vi "MC-21C Driver_query.vi"(0 "Peristaltic Pump COM":refnum<visa-resource-name>="COM3", 1 "Speed (rpm)":string, 5 "Operation":T1(ring), 7 "Address":u8, 9 "Set address (0-255)":u8, 12 "Step":string) -> (6 "PerisPump running":bool, 10 "Write buffer":string, 15 "Read buffer":string)   [LabVIEW 2023]
panel:
  out "Current address":u8
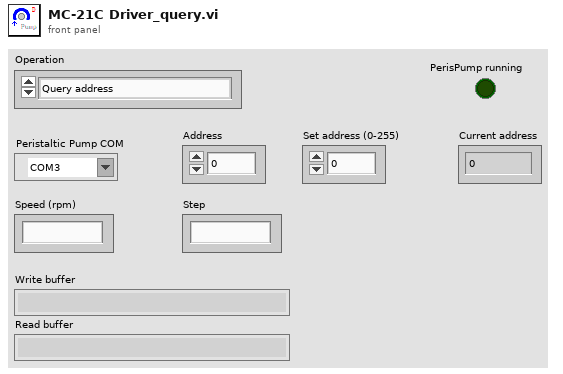
[diagram p1: front panel]
types:
  T1 = enum16{"Query address", "Set address", "Set speed", "Clockwise rotation", "Counterclockwise rotation", "Stop"}
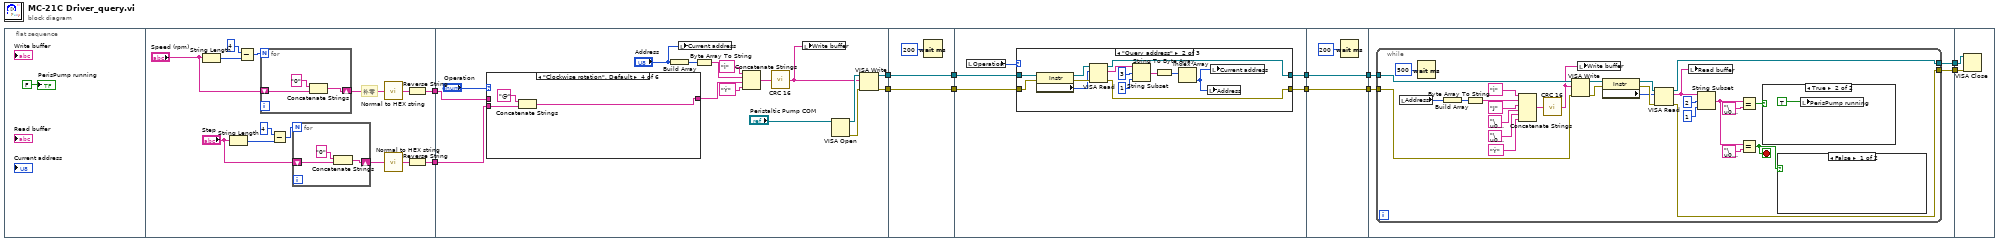
[diagram p0: block diagram]
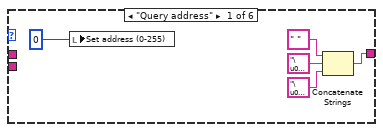
[diagram p2: hidden frame]
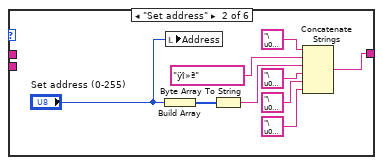
[diagram p3: hidden frame]
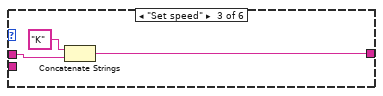
[diagram p4: hidden frame]
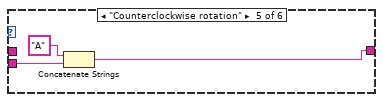
[diagram p5: hidden frame]
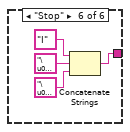
[diagram p6: hidden frame]
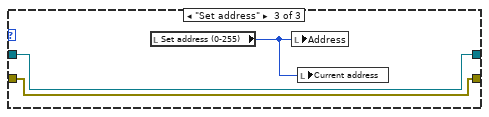
[diagram p8: hidden frame]
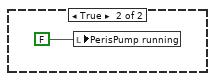
[diagram p10: hidden frame]
diagram:
  n1 = flat-sequence {
    tunnel: [w21] -> w11
    tunnel: [w14] -> w12
    tunnel: [w42] -> w6
    tunnel: [w41] -> w4
    tunnel: w12 -> [w40]
    tunnel: w11 -> [w39]
    tunnel: w6 -> [w79]
    tunnel: [w79] -> w5
    tunnel: w4 -> [w78]
    tunnel: [w78] -> w3
    tunnel: w5 -> [w83]
    tunnel: [w81] -> w8
    tunnel: w3 -> [w82]
    tunnel: [w80] -> w7
    tunnel: w8 -> [w105]
    tunnel: [w105] -> w10
    tunnel: w7 -> [w104]
    tunnel: [w104] -> w9
    tunnel: w10 -> [w109]
    tunnel: w9 -> [w108]
    tunnel: [w107] -> w2
    tunnel: [w106] -> w1
    tunnel: w2 -> [w141]
    tunnel: w1 -> [w140]
    frame #0 {
      "PerisPump running" <- FALSE ("PerisPump running")
    }
    frame #1 {
      # "补零"
      n2 = String Length(string="Speed (rpm)") -> (length=w25:i32)
      n3 = String Length(string="Step") -> (length=w19:i32)
      n4 = Subtract(x=4, y=w25) -> (x-y=w27:i32)
      n5 = for {
        N: w27 -> [_]
        shift-right: [w31] -> w23
        shift-left: "Speed (rpm)" -> [w33]
        n6 = Concatenate Strings("0" ("string"), w33) -> (w31:string)
      }
      n7 = Subtract(x=4, y=w19) -> (x-y=w18:i32)
      n8 = for {
        N: w18 -> [_]
        shift-right: [w28] -> w16
        shift-left: "Step" -> [w30]
        n9 = Concatenate Strings("0" ("string"), w30) -> (w28:string)
      }
      n10 = call "Normal to HEX string.vi"("input normal string"=w23) -> ("output HEX string"=w22:string)
      n11 = call "Normal to HEX string.vi"("input normal string"=w16) -> ("output HEX string"=w20:string)
      n12 = Reverse String(1:w22) -> (0:w21:string)
      n13 = Reverse String(1:w20) -> (0:w14:string)
    }
    frame #2 {
      n14 = case shown="\"Clockwise rotation\", Default" "Operation" {
        tunnel: [w50 w58 w65 w68 w71 w73] -> w46
        tunnel: w40 -> [_ _ _ w67 w70 _]
        tunnel: w39 -> [_ _ w64 _ _ _]
        frame "Query address" {
          n15 = local write "Set address (0-255)"(u8 0 ("Address (0-255)")) -> ()
          n16 = Concatenate Strings(" " ("string"), "\u0000" ("string"), "\u0000" ("string")) -> (w50:string)
        }
        frame "Set address" {
          n17 = Build Array("Set address (0-255)") -> (w57:u8[])
          n18 = local write "Address"("Set address (0-255)") -> ()
          n19 = Byte Array To String(unsigned byte array=w57) -> (string=w56:string)
          n20 = Concatenate Strings("\u0000" ("string"), "ÿî»ª" ("string"), w56, "\u0000" ("string"), "\u0000" ("string"), "\u0000" ("string")) -> (w58:string)
        }
        frame "Set speed" {
          n21 = Concatenate Strings("K" ("string"), w64) -> (w65:string)
        }
        frame "Clockwise rotation", Default {
          n22 = Concatenate Strings("@" ("string"), w67) -> (w68:string)
        }
        frame "Counterclockwise rotation" {
          n23 = Concatenate Strings("A" ("string"), w70) -> (w71:string)
        }
        frame "Stop" {
          n24 = Concatenate Strings("I" ("string"), "\u0000" ("string"), "\u0000" ("string")) -> (w73:string)
        }
      }
      n25 = Build Array("Address") -> (w38:u8[])
      n26 = local write "Current address"("Address") -> ()
      n27 = Byte Array To String(unsigned byte array=w38) -> (string=w37:string)
      n28 = Concatenate Strings("Ì" ("string"), w37, w46, "Ý" ("string")) -> (w36:string)
      n29 = call "CRC 16.vi"("input HEX string"=w36) -> ("output HEX string"=w35:string)
      n30 = local write "Write buffer"(w35) -> ()
      n31 = VISA Open(VISA resource name="Peristaltic Pump COM") -> (VISA resource name=w45:refnum<visa-resource-name>, error out=w44:errorcluster)  [unwired: 4 in]
      n32 = VISA Write(VISA resource name=w45, write buffer=w35, error in (no error)=w44) -> (VISA resource name out=w42:refnum<visa-resource-name>, error out=w41:errorcluster)  [unwired: 1 out]
    }
    frame #3 {
      n33 = Wait (ms)(milliseconds to wait=u32 200) -> ()  [unwired: 1 out]
    }
    frame #4 {
      n34 = local read "Operation"() -> (w84:T1)
      n35 = case shown="\"Query address\"" w84 {
        tunnel: w83 -> [w86 w96 w102]
        tunnel: w82 -> [w85 w95 w101]
        tunnel: [w86 w89 w102] -> w81
        tunnel: [w85 w88 w101] -> w80
        frame "Set speed", Default {
        }
        frame "Query address" {
          n36 = property class="Instr"(reference=w96, error in=w95) -> (reference out=w99:refnum<visa-resource-name>, error out=w98:errorcluster, "Serial Settings:Number of Bytes at Serial Port"=w97:u32)
          n37 = VISA Read(VISA resource name=w99, byte count=w97, error in (no error)=w98) -> (VISA resource name out=w89:refnum<visa-resource-name>, read buffer=w92:string, error out=w88:errorcluster)  [unwired: 1 out]
          n38 = String Subset(string=w92, offset (0)=3, length (rest)=1 ("length (rest)")) -> (substring=w91:string)
          n39 = String To Byte Array(string=w91) -> (unsigned byte array=w90:u8[])
          n40 = Index Array(array=w90) -> (element=w87:u8)  [unwired: 1 in]
          n41 = local write "Address"(w87) -> ()
          n42 = local write "Current address"(w87) -> ()
        }
        frame "Set address" {
          n43 = local read "Set address (0-255)"() -> (w100:u8)
          n44 = local write "Address"(w100) -> ()
          n45 = local write "Current address"(w100) -> ()
        }
      }
    }
    frame #5 {
      n46 = Wait (ms)(milliseconds to wait=u32 200) -> ()  [unwired: 1 out]
    }
    frame #6 {
      n47 = while {
        tunnel: w109 -> [w128]
        tunnel: w108 -> [w127]
        tunnel: [w124] -> w107
        tunnel: [w123] -> w106
        stop <- w114 stop-if-true
        n48 = local read "Address"() -> (w132:u8)
        n49 = Wait (ms)(milliseconds to wait=u32 500) -> ()  [unwired: 1 out]
        n50 = Build Array(w132) -> (w133:u8[])
        n51 = Byte Array To String(unsigned byte array=w133) -> (string=w131:string)
        n52 = Concatenate Strings("Ì" ("string"), w131, "J" ("string"), "\u0000" ("string"), "\u0000" ("string"), "Ý" ("string")) -> (w117:string)
        n53 = call "CRC 16.vi"("input HEX string"=w117) -> ("output HEX string"=w116:string)
        n54 = VISA Write(VISA resource name=w128, write buffer=w116, error in (no error)=w127) -> (VISA resource name out=w122:refnum<visa-resource-name>, error out=w121:errorcluster)  [unwired: 1 out]
        n55 = local write "Write buffer"(w116) -> ()
        n56 = property class="Instr"(reference=w122, error in=w121) -> (reference out=w120:refnum<visa-resource-name>, error out=w119:errorcluster, "Serial Settings:Number of Bytes at Serial Port"=w118:u32)
        n57 = VISA Read(VISA resource name=w120, byte count=w118, error in (no error)=w119) -> (VISA resource name out=w124:refnum<visa-resource-name>, read buffer=w115:string, error out=w123:errorcluster)  [unwired: 1 out]
        n58 = local write "Read buffer"(w115) -> ()
        n59 = String Subset(string=w115, offset (0)=2, length (rest)=1 ("length (rest)")) -> (substring=w112:string)
        n60 = Equal?(x=w112, y="\u0004") -> (x = y?=w110:bool)
        n61 = Equal?(x=w112, y="\u0000") -> (x = y?=w114:bool)
        n62 = case shown="True" w110 {
          frame False {
          }
          frame True {
            n63 = local write "PerisPump running"(TRUE ("PerisPump running")) -> ()
          }
        }
        n64 = case shown="False" w114 {
          frame False {
          }
          frame True {
            n65 = local write "PerisPump running"(FALSE ("PerisPump running")) -> ()
          }
        }
      }
    }
    frame #7 {
      n66 = VISA Close(VISA resource name=w141, error in (no error)=w140) -> ()  [unwired: 1 out]
    }
  }
